vi "TCam_PointCalculator.vi"(10 "Cluster":T1={"Core"={"Current VI Reference"=refnum, "Close Panel on Exit?"=FALSE}, "Image Out"=refnum, "State"=0, "Points"={"Top Left"={"X"=0.0, "Y"=0.0}, "Top Right"={"X"=0.0, "Y"=0.0}, "Bottom Left"={"X"=0.0, "Y"=0.0}, "Bottom Right"={"X"=0.0, "Y"=0.0}, "x space 2"=0.0, "y space 2"=0.0, "x_space"=0.0, "y_space"=0.0, "Pixels"=[], "Fixpoint"={"X"=0.0, "Y"=0.0}}, "img_array"=[], "Temps"=[], "Temps_Array"=[], "Scan Area"=0.0, "Fixpoint Area"=0.0, "Config"={"Freezing"={"Cutoff"=2.0, "EndIndex"=2}}, "PCR Size"=0, "ImageCount"=0, "ShowGradient"=FALSE} {"Points"."Bottom Right"."Y" format="%.2f"; "Points"."Bottom Right"."X" format="%.2f"; "Points"."Top Left"."Y" format="%.2f"; "Points"."Top Left"."X" format="%.2f"; "Points"."Top Right"."Y" format="%.2f"; "Points"."Top Right"."X" format="%.2f"; "Points"."Bottom Left"."Y" format="%.2f"; "Points"."Bottom Left"."X" format="%.2f"; "Points"."Fixpoint"."Y" format="%.2f"; "Points"."Fixpoint"."X" format="%.2f"}, 11 "Size":u16) -> (3 "Points":T3[](array[typedef]) {"Y" format="%.2f"; "X" format="%.2f"})   [LabVIEW 2022 SP3]
uses:
  DataCluster_TCAL.ctl
  <vilib>/vision/Image Controls.llb/IMAQ Image.ctl
  TCE_Config.ctl
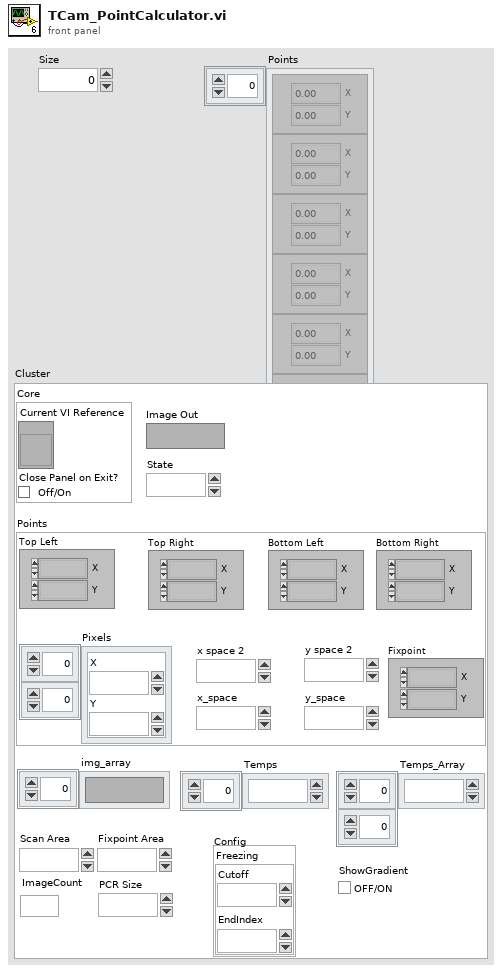
[diagram p1: front panel]
types:
  T1 = typedef "DataCluster_TCAL.ctl" = cluster{"Core":cluster{"Current VI Reference":refnum<vi>, "Close Panel on Exit?":bool}, "Image Out":T2, "State":i32, "Points":cluster{"Top Left":T3, "Top Right":T3, "Bottom Left":T3, "Bottom Right":T3, "x space 2":dbl, "y space 2":sgl, "x_space":sgl, "y_space":sgl, "Pixels":cluster{"X":i32, "Y":i32}[][], "Fixpoint":T3}, "img_array":T2[], "Temps":dbl[], "Temps_Array":dbl[][], "Scan Area":dbl, "Fixpoint Area":dbl, "Config":T4, "PCR Size":u16, "ImageCount":i32, "ShowGradient":bool}
  T2 = typedef "IMAQ Image.ctl" = refnum<image>
  T3 = typedef "IMAQ Point" = cluster{"X":sgl, "Y":sgl}
  T4 = typedef "TCE_Config.ctl" = cluster{"Freezing":cluster{"Cutoff":dbl, "EndIndex":i32}}
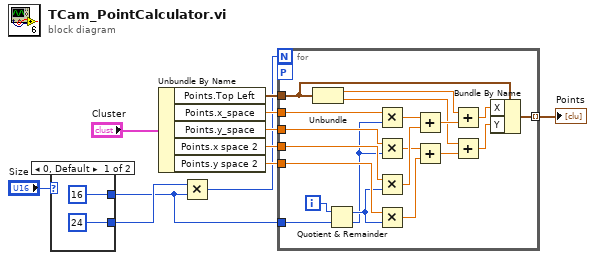
[diagram p0: block diagram]
diagram:
  n1 = case shown="0, Default" "Size" {
    tunnel: [24 _] -> w11
    tunnel: [16 _] -> w1
    frame 0, Default {
    }
    frame 1 {
    }
  }
  n2 = Unbundle By Name("Cluster") -> ("Points.Top Left"=w4:T3, "Points.x_space"=w5:sgl, "Points.y_space"=w7:sgl, "Points.x space 2"=w6:dbl, "Points.y space 2"=w8:sgl)
  n3 = Multiply(x=w11, y=w1) -> (x*y=w3:i32)
  n4 = for {
    N: w3 -> [_]
    tunnel: w4 -> [w25]
    tunnel: w5 -> [w32]
    tunnel: w1 -> [w29]
    tunnel: w6 -> [w28]
    tunnel: w7 -> [w21]
    tunnel: w8 -> [w16]
    tunnel: [w17] -> w9 mode=indexing
    workers-P: _ -> [_]
    i -> [w30]
    n5 = Unbundle(w25) -> ("X"=w33:sgl, "Y"=w22:sgl)
    n6 = Quotient & Remainder(x=w30, y=w29) -> (x-y*floor(x/y)=w15:i32, floor(x/y)=w14:i32)
    n7 = Multiply(x=w32, y=w14) -> (x*y=w31:sgl)
    n8 = Multiply(x=w21, y=w14) -> (x*y=w20:sgl)
    n9 = Multiply(x=w28, y=w15) -> (x*y=w26:dbl)
    n10 = Multiply(x=w16, y=w15) -> (x*y=w18:sgl)
    n11 = Add(x=w31, y=w26) -> (x+y=w27:dbl)
    n12 = Add(x=w20, y=w18) -> (x+y=w19:sgl)
    n13 = Add(x=w33, y=w27) -> (x+y=w24:dbl)
    n14 = Add(x=w22, y=w19) -> (x+y=w23:sgl)
    n15 = Bundle By Name(cluster=w25, "X"=w24, "Y"=w23) -> (w17:T3)
  }
  "Points" <- w9
